vi "Light Page.vi"() -> ()   [LabVIEW 2020, in "3D Plot.lvclass"]
uses:
  <vilib>/Math Plots/3D Math Plots/3D Plot/3D Plot/3D Plot.lvclass
  <vilib>/Math Plots/3D Math Plots/3D Plot/3D Plot/Typedef/Light Property.ctl
  <vilib>/Math Plots/3D Math Plots/3D Plot/3D Plot/Typedef/Light Specific.ctl
  <vilib>/Math Plots/3D Math Plots/3D Plot/3D Plot/Typedef/Dialog State.ctl
  <vilib>/Math Plots/3D Math Plots/3D Plot/3D Plot/Typedef/Temp Scene State.ctl
  <vilib>/Math Plots/3D Math Plots/3D Plot/3D Plot/Typedef/Temp Scene Property Action.ctl
panel:
  in  "Distance":sgl(slide) scale=0.0..20.0
  in  "Latitude":sgl(slide) min=0 max=360 scale=0.0..360.0
  in  "Longitude":sgl(slide) min=0 max=360 scale=0.0..360.0
  in  "Enable Light":bool caption="Enable light"
  in  "Attenuation":u16(ring) items=["None ", "Linear", "Quadratic"]
  in  "Light Color":u32(colorbox) caption="Light color"
  in  "Light List":i32(listbox) caption="Light list"
  in  "Enable Lighting":bool caption="Enable lighting"
  in  "Event Registration":refnum<event-registration>
  out "Light Property Out":T1
  in  "Light Property In":T1
  # "Light"
  # "Single Light"
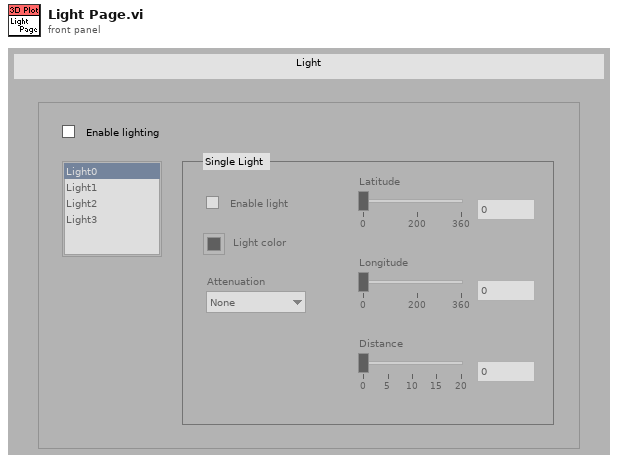
[diagram p1: front panel]
types:
  T1 = typedef "3D Plot.lvclass/Light Property.ctl" = cluster{"Enable Lighting?":bool, "Ambient Color":u32, "Light Array":T2[]}
  T2 = typedef "3D Plot.lvclass/Light Specific.ctl" = cluster{"Enable Light?":bool, "Light Color":u32, "Light Latitude":sgl, "Light Longitude":sgl, "Light Distance":sgl, "Attenuation":enum16{"None", "Linear", "Quadratic"}}
  T3 = typedef "3D Plot.lvclass/Dialog State.ctl" = enum16{"Initialize", "Read Porperty", "Write Property", "Idle", "Exit"}
  T4 = typedef "3D Plot.lvclass/Temp Scene Property Action.ctl" = enum16{"Graph Property", "Light Property", "Axis Property", "Value Pair Property", "Format Property", "Cursor Property", "Plot Specific Property"}
  T5 = typedef "3D Plot.lvclass/Temp Scene State.ctl" = enum16{"Create", "Update Scene", "Get Plot Representation", "Destory"}
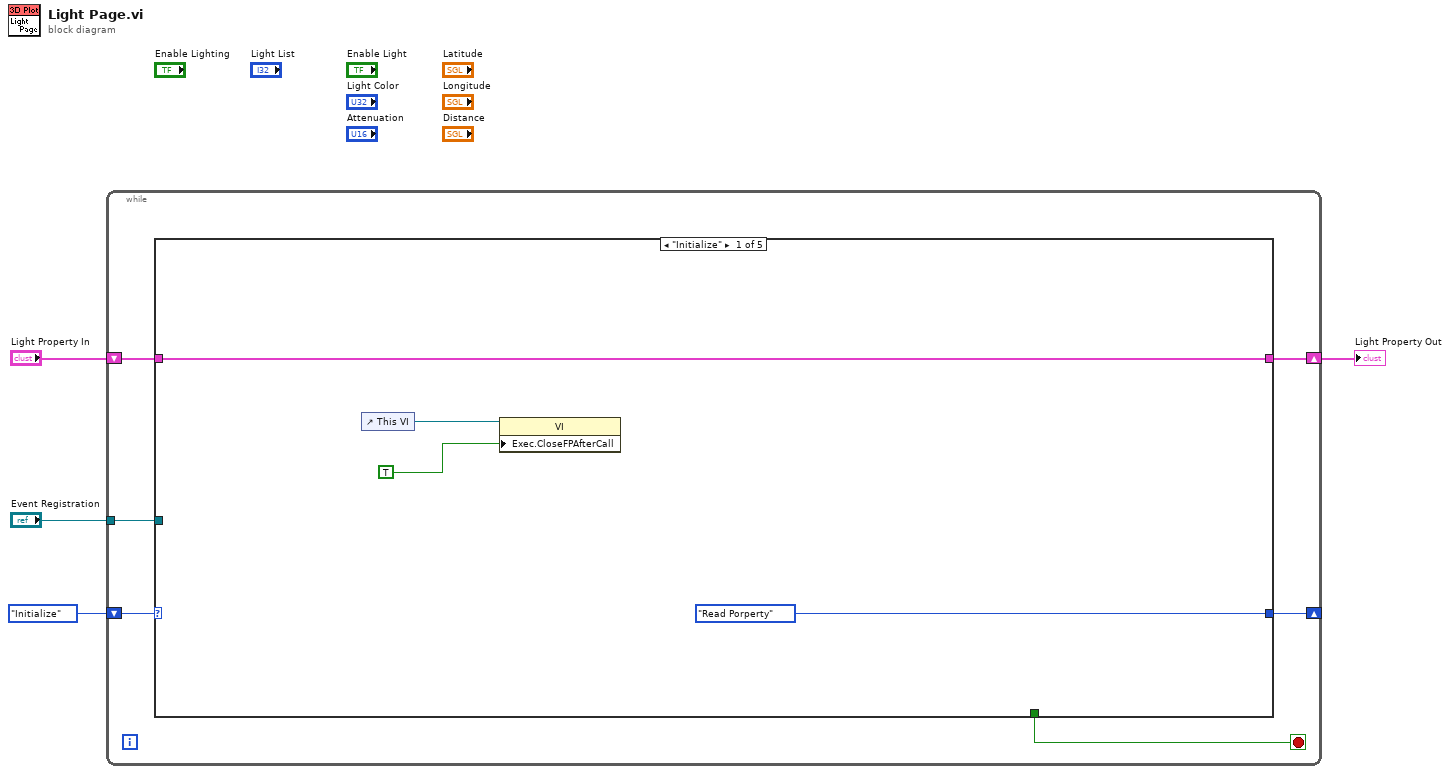
[diagram p0: block diagram]
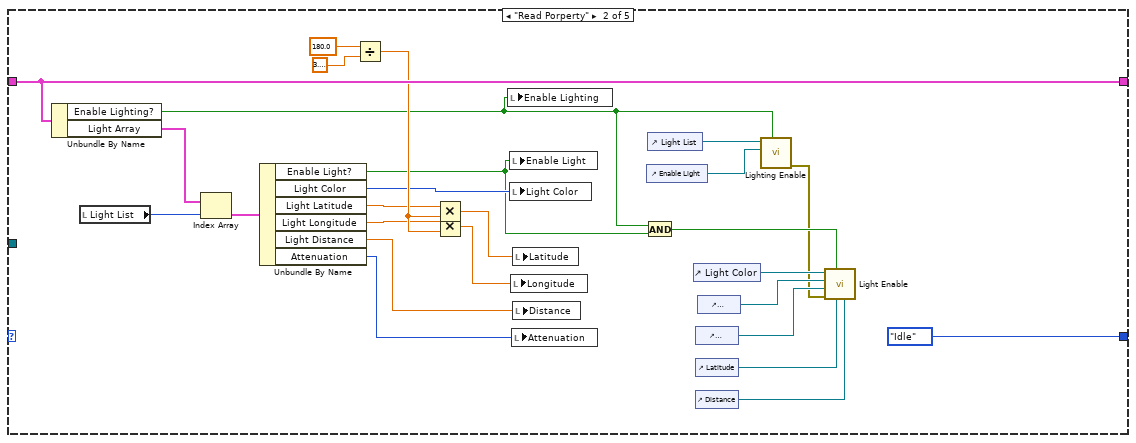
[diagram p2: hidden frame]
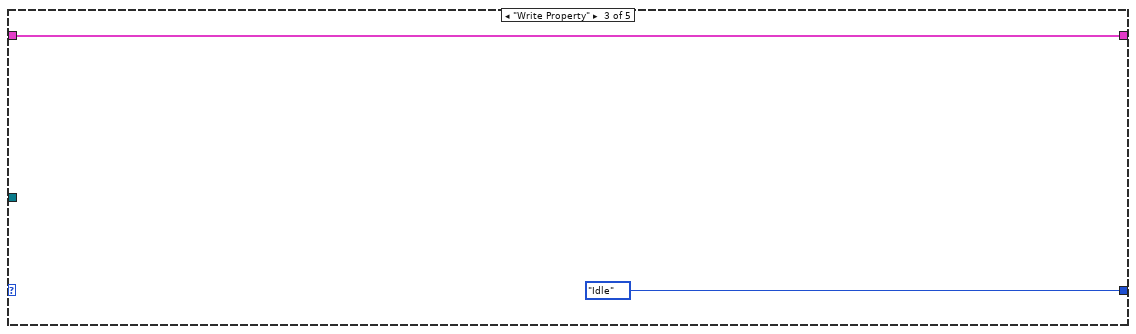
[diagram p3: hidden frame]
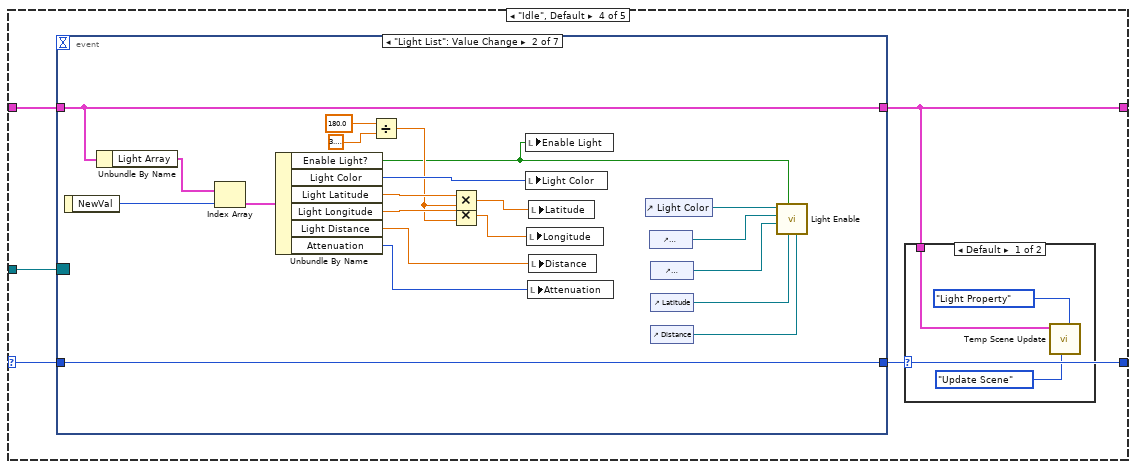
[diagram p4: hidden frame]
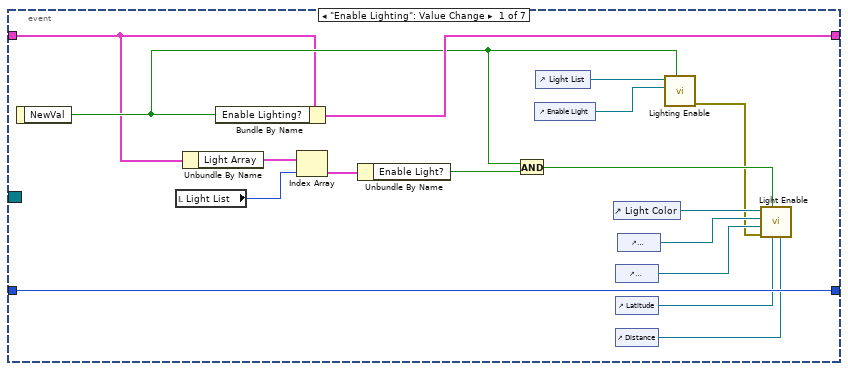
[diagram p6: hidden frame]
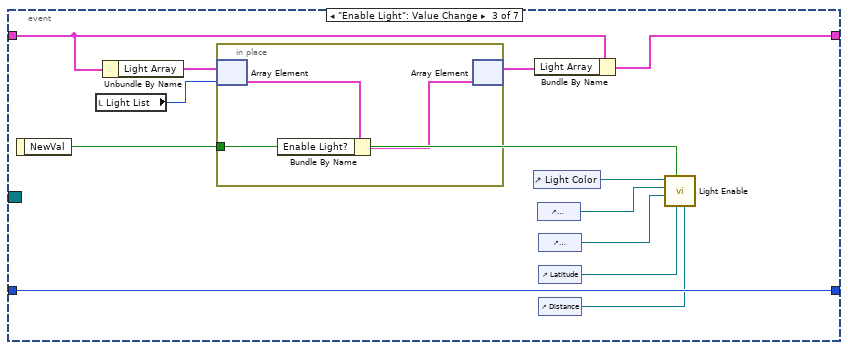
[diagram p7: hidden frame]
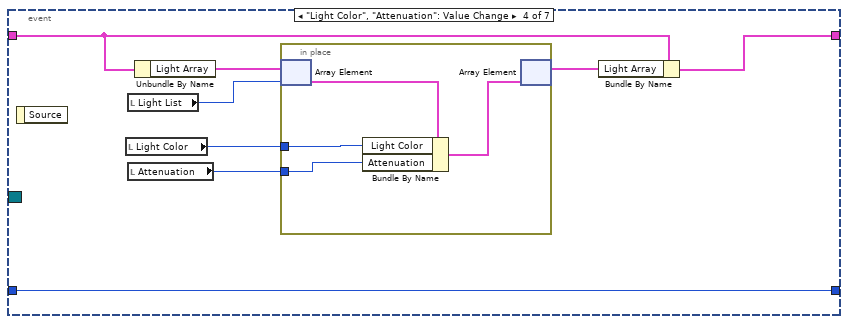
[diagram p8: hidden frame]
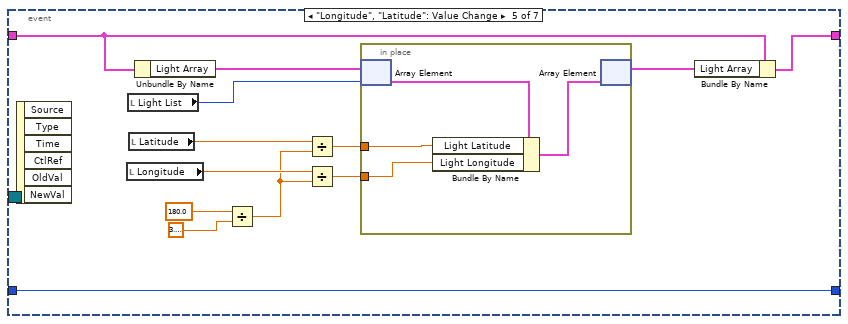
[diagram p9: hidden frame]
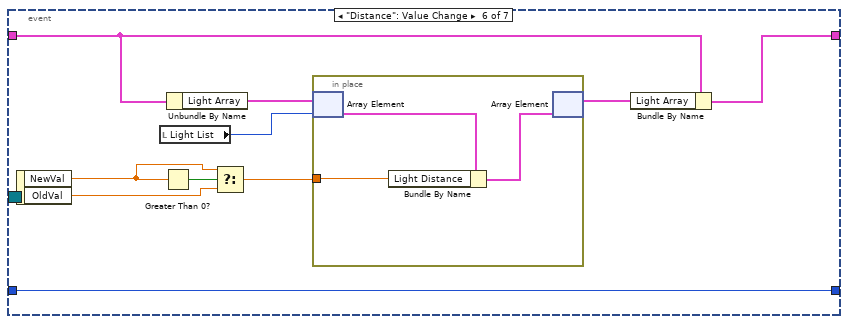
[diagram p10: hidden frame]
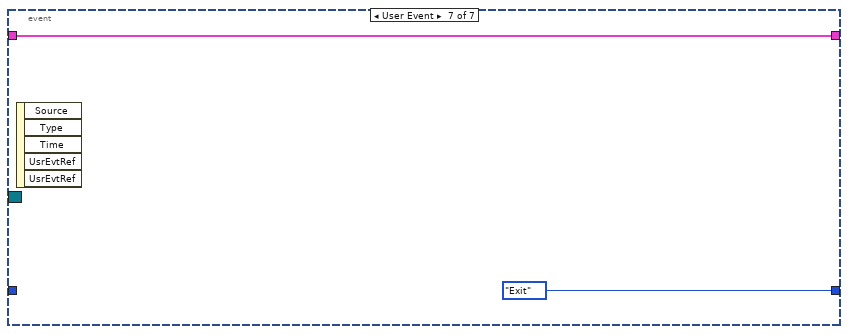
[diagram p11: hidden frame]
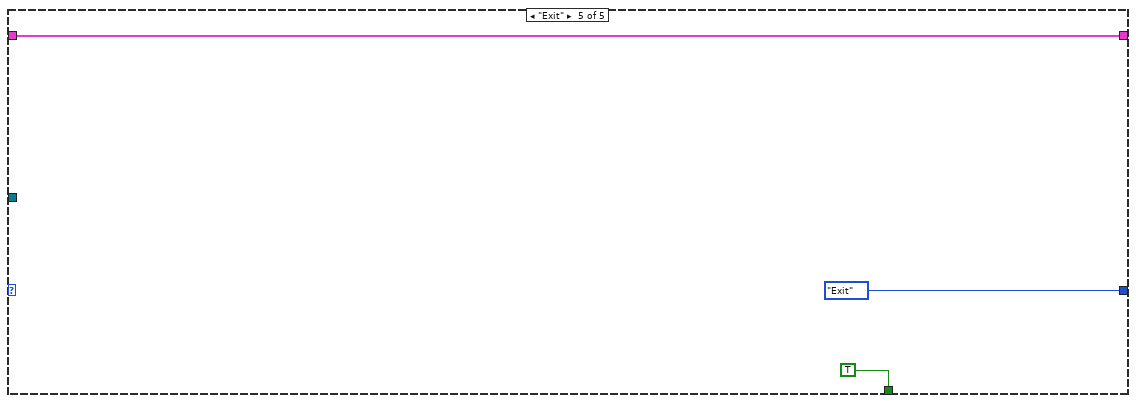
[diagram p12: hidden frame]
diagram:
  n1 = while {
    shift-right: [w9] -> w3
    shift-left: "Light Property In" -> [w10]
    shift-right: [w5] -> _
    shift-left: Dialog_State."Initialize" ("Enum") -> [w6]
    tunnel: "Event Registration" -> [w7]
    stop <- w8 stop-if-true
    n2 = case shown="\"Initialize\"" w6 {
      selector: w6 -> [_ _ _ w45 _]
      tunnel: w10 -> [w14 w40 w41 w47 w148]
      tunnel: [w14 w40 w41 w44 w148] -> w9
      tunnel: [Dialog_State."Read Porperty" ("Enum") Dialog_State."Idle" Dialog_State."Idle" w43 Dialog_State."Exit"] -> w5
      tunnel: [_ _ _ _ TRUE] -> w8
      tunnel: w7 -> [_ _ _ w46 _]
      frame "Initialize" {
        n3 = control-ref of="This VI"() -> (w13:refnum<vi>)
        n4 = property class="VI"(reference=w13, "Exec.CloseFPAfterCall"=TRUE ("Execution:Close After Call")) -> ()  [unwired: 1 in, 2 out]
      }
      frame "Read Porperty" {
        n5 = Unbundle By Name(w40) -> ("Enable Lighting?"=w20:bool, "Light Array"=w35:T2[])
        n6 = local read "Light List"() -> (w34:i32)
        n7 = Index Array(array=w35, index=w34) -> (element=w33:T2)
        n8 = Unbundle By Name(w33) -> ("Enable Light?"=w19:bool, "Light Color"=w28:u32, "Light Latitude"=w32:sgl, "Light Longitude"=w31:sgl, "Light Distance"=w27:sgl, "Attenuation"=w26:enum16{"None", "Linear", "Quadratic"})
        n9 = Divide(x=sgl 180.0, y=sgl 3.1415927) -> (x/y=w38:sgl)
        n10 = Multiply(x=w32, y=w38) -> (x*y=w30:sgl)
        n11 = Multiply(x=w31, y=w38) -> (x*y=w29:sgl)
        n12 = local write "Enable Lighting"(w20) -> ()
        n13 = local write "Enable Light"(w19) -> ()
        n14 = local write "Light Color"(w28) -> ()
        n15 = local write "Longitude"(w29) -> ()
        n16 = local write "Attenuation"(w26) -> ()
        n17 = local write "Latitude"(w30) -> ()
        n18 = local write "Distance"(w27) -> ()
        n19 = And(x=w20, y=w19) -> (x .and. y?=w18:bool)
        n20 = control-ref of="Enable Light"() -> (w16:refnum<vi>)
        n21 = control-ref of="Light List"() -> (w17:refnum<vi>)
        n22 = control-ref of="Light Color"() -> (w25:refnum<vi>)
        n23 = control-ref of="Longitude"() -> (w23:refnum<vi>)
        n24 = control-ref of="Latitude"() -> (w22:refnum<vi>)
        n25 = control-ref of="Distance"() -> (w21:refnum<vi>)
        n26 = control-ref of="Attenuation"() -> (w24:refnum<vi>)
        n27 = call <vilib>:"Lighting Enable.vi"("Enabled?"=w20, "Enable light Refnum"=w16, "Light List Refnum"=w17) -> ("error out"=w15:errorcluster)  [unwired: 2 in, 6 out]
        n28 = call <vilib>:"Light Enable.vi"("Distance Refnum"=w21, "Latitude Refnum"=w22, "Enabled?"=w18, "error in (no error)"=w15, "Longitude Refnum"=w23, "Attenuation Refnum"=w24, "Light color Refnum"=w25) -> ()  [unwired: 5 out]
      }
      frame "Write Property" {
      }
      frame "Idle", Default {
        n29 = event shown="[1] \"Light List\": Value Change" {
          selector: w46 -> [_ _ _ _ _ _ _]
          dyn-events: _ -> [_ _ _ _ _ _ _]
          timeout: _ -> [_ _ _ _ _ _ _]
          tunnel: w47 -> [w56 w68 w97 w107 w124 w141 w147]
          tunnel: [w67 w68 w96 w108 w125 w140 w147] -> w44
          tunnel: [w66 w88 w100 w111 w128 w133 Dialog_State."Exit"] -> w43
          tunnel: w45 -> [w66 w88 w100 w111 w128 w133 _]
          event "Enable Lighting": Value Change {
            n30 = event-data() -> ("NewVal"=w59:bool)  [unwired: 1 out]
            n31 = local read "Light List"() -> (w58:i32)
            n32 = Unbundle By Name(w56) -> ("Light Array"=w55:T2[])
            n33 = Bundle By Name(cluster=w56, "Enable Lighting?"=w59) -> (w67:T1)
            n34 = Index Array(array=w55, index=w58) -> (element=w57:T2)
            n35 = Unbundle By Name(w57) -> ("Enable Light?"=w54:bool)
            n36 = And(x=w59, y=w54) -> (x .and. y?=w60:bool)
            n37 = control-ref of="Enable Light"() -> (w52:refnum<vi>)
            n38 = control-ref of="Light List"() -> (w53:refnum<vi>)
            n39 = control-ref of="Light Color"() -> (w65:refnum<vi>)
            n40 = control-ref of="Longitude"() -> (w63:refnum<vi>)
            n41 = control-ref of="Latitude"() -> (w62:refnum<vi>)
            n42 = control-ref of="Distance"() -> (w61:refnum<vi>)
            n43 = control-ref of="Attenuation"() -> (w64:refnum<vi>)
            n44 = call <vilib>:"Lighting Enable.vi"("Enabled?"=w59, "Enable light Refnum"=w52, "Light List Refnum"=w53) -> ("error out"=w51:errorcluster)  [unwired: 2 in, 6 out]
            n45 = call <vilib>:"Light Enable.vi"("Distance Refnum"=w61, "Latitude Refnum"=w62, "Enabled?"=w60, "error in (no error)"=w51, "Longitude Refnum"=w63, "Attenuation Refnum"=w64, "Light color Refnum"=w65) -> ()  [unwired: 5 out]
          }
          event "Light List": Value Change {
            n46 = event-data() -> ("NewVal"=w69:i32)  [unwired: 1 out]
            n47 = Unbundle By Name(w68) -> ("Light Array"=w75:T2[])
            n48 = Index Array(array=w75, index=w69) -> (element=w87:T2)
            n49 = Unbundle By Name(w87) -> ("Enable Light?"=w70:bool, "Light Color"=w82:u32, "Light Latitude"=w86:sgl, "Light Longitude"=w85:sgl, "Light Distance"=w81:sgl, "Attenuation"=w80:enum16{"None", "Linear", "Quadratic"})
            n50 = Divide(x=sgl 180.0, y=sgl 3.1415927) -> (x/y=w72:sgl)
            n51 = Multiply(x=w86, y=w72) -> (x*y=w84:sgl)
            n52 = Multiply(x=w85, y=w72) -> (x*y=w83:sgl)
            n53 = local write "Enable Light"(w70) -> ()
            n54 = local write "Light Color"(w82) -> ()
            n55 = local write "Longitude"(w83) -> ()
            n56 = local write "Attenuation"(w80) -> ()
            n57 = local write "Latitude"(w84) -> ()
            n58 = local write "Distance"(w81) -> ()
            n59 = control-ref of="Light Color"() -> (w79:refnum<vi>)
            n60 = control-ref of="Attenuation"() -> (w78:refnum<vi>)
            n61 = control-ref of="Longitude"() -> (w77:refnum<vi>)
            n62 = control-ref of="Latitude"() -> (w76:refnum<vi>)
            n63 = control-ref of="Distance"() -> (w71:refnum<vi>)
            n64 = call <vilib>:"Light Enable.vi"("Distance Refnum"=w71, "Latitude Refnum"=w76, "Enabled?"=w70, "Longitude Refnum"=w77, "Attenuation Refnum"=w78, "Light color Refnum"=w79) -> ()  [unwired: 1 in, 5 out]
          }
          event "Enable Light": Value Change {
            n65 = event-data() -> ("NewVal"=w89:bool)  [unwired: 1 out]
            n66 = local read "Light List"() -> (w98:i32)
            n67 = Unbundle By Name(w97) -> ("Light Array"=w99:T2[])
            n68 = in-place {
              in-place-border: w89 -> [w101]
              n69 = in-place-array #1(w99, w98) -> (w103:T2)
              n70 = Bundle By Name(cluster=w103, "Enable Light?"=w101) -> (w102:T2)
              n71 = in-place-array #1(w102) -> (w95:T2[])  [unwired: 1 out]
            }
            n72 = control-ref of="Light Color"() -> (w94:refnum<vi>)
            n73 = Bundle By Name(cluster=w97, "Light Array"=w95) -> (w96:T1)
            n74 = control-ref of="Attenuation"() -> (w93:refnum<vi>)
            n75 = control-ref of="Longitude"() -> (w92:refnum<vi>)
            n76 = control-ref of="Latitude"() -> (w91:refnum<vi>)
            n77 = control-ref of="Distance"() -> (w90:refnum<vi>)
            n78 = call <vilib>:"Light Enable.vi"("Distance Refnum"=w90, "Latitude Refnum"=w91, "Enabled?"=w89, "Longitude Refnum"=w92, "Attenuation Refnum"=w93, "Light color Refnum"=w94) -> ()  [unwired: 1 in, 5 out]
          }
          event "Light Color", "Attenuation": Value Change {
            n79 = event-data() -> ()  [unwired: 2 out]
            n80 = local read "Light Color"() -> (w106:u32)
            n81 = local read "Light List"() -> (w109:i32)
            n82 = local read "Attenuation"() -> (w105:u16)
            n83 = Unbundle By Name(w107) -> ("Light Array"=w110:T2[])
            n84 = in-place {
              in-place-border: w106 -> [w113]
              in-place-border: w105 -> [w112]
              n85 = in-place-array #2(w110, w109) -> (w115:T2)
              n86 = Bundle By Name(cluster=w115, "Light Color"=w113, "Attenuation"=w112) -> (w114:T2)
              n87 = in-place-array #2(w114) -> (w104:T2[])  [unwired: 1 out]
            }
            n88 = Bundle By Name(cluster=w107, "Light Array"=w104) -> (w108:T1)
          }
          event "Longitude", "Latitude": Value Change {
            n89 = event-data() -> ()  [unwired: 7 out]
            n90 = local read "Longitude"() -> (w118:sgl)
            n91 = local read "Light List"() -> (w126:i32)
            n92 = local read "Latitude"() -> (w120:sgl)
            n93 = Unbundle By Name(w124) -> ("Light Array"=w127:T2[])
            n94 = Divide(x=sgl 180.0, y=sgl 3.1415927) -> (x/y=w117:sgl)
            n95 = Divide(x=w120, y=w117) -> (x/y=w119:sgl)
            n96 = Divide(x=w118, y=w117) -> (x/y=w116:sgl)
            n97 = in-place {
              in-place-border: w119 -> [w130]
              in-place-border: w116 -> [w129]
              n98 = in-place-array #3(w127, w126) -> (w132:T2)
              n99 = Bundle By Name(cluster=w132, "Light Latitude"=w130, "Light Longitude"=w129) -> (w131:T2)
              n100 = in-place-array #3(w131) -> (w123:T2[])  [unwired: 1 out]
            }
            n101 = Bundle By Name(cluster=w124, "Light Array"=w123) -> (w125:T1)
          }
          event "Distance": Value Change {
            n102 = event-data() -> ("NewVal"=w137:sgl, "OldVal"=w136:sgl)  [unwired: 1 out]
            n103 = local read "Light List"() -> (w134:i32)
            n104 = Greater Than 0?(x=w137) -> (x > 0?=w142:bool)
            n105 = Unbundle By Name(w141) -> ("Light Array"=w139:T2[])
            n106 = Select(t=w137, s=w142, f=w136) -> (s? t:f=w135:sgl)
            n107 = in-place {
              in-place-border: w135 -> [w143]
              n108 = in-place-array #4(w139, w134) -> (w145:T2)
              n109 = Bundle By Name(cluster=w145, "Light Distance"=w143) -> (w144:T2)
              n110 = in-place-array #4(w144) -> (w138:T2[])  [unwired: 1 out]
            }
            n111 = Bundle By Name(cluster=w141, "Light Array"=w138) -> (w140:T1)
          }
          event User Event {
            n112 = event-data() -> ()  [unwired: 6 out]
          }
        }
        n113 = case shown="Default" w43 {
          tunnel: w44 -> [w49 _]
          frame Default {
            n114 = call <vilib>:"Temp Scene Update.vi"("Property Name"=Temp_Scene_Property_Action."Light Property", "State"=Temp_Scene_State."Update Scene", "Property In"=w49) -> ()  [unwired: 3 in, 6 out]
          }
          frame "Exit" {
          }
        }
      }
      frame "Exit" {
      }
    }
  }
  "Light Property Out" <- w3
